vi "IMAQController.CalculateOverlay.vi"(1 "activatedCameras":T2(array[cluster]), 2 "Select Camera":u16(ring) items=["HITRAP TR1DF0", "HITRAP TR1DF2"], 6 "Line Every mm":dbl=10.0) -> (16 "Overlay Lines":T3(array[cluster]), 18 "Error?":bool)   [LabVIEW 2014, in "IMAQController.lvlib"]
uses:
  IMAQController.lvlib
  <vilib>/Utility/miscctls.llb/LVPoint32TypeDef.ctl
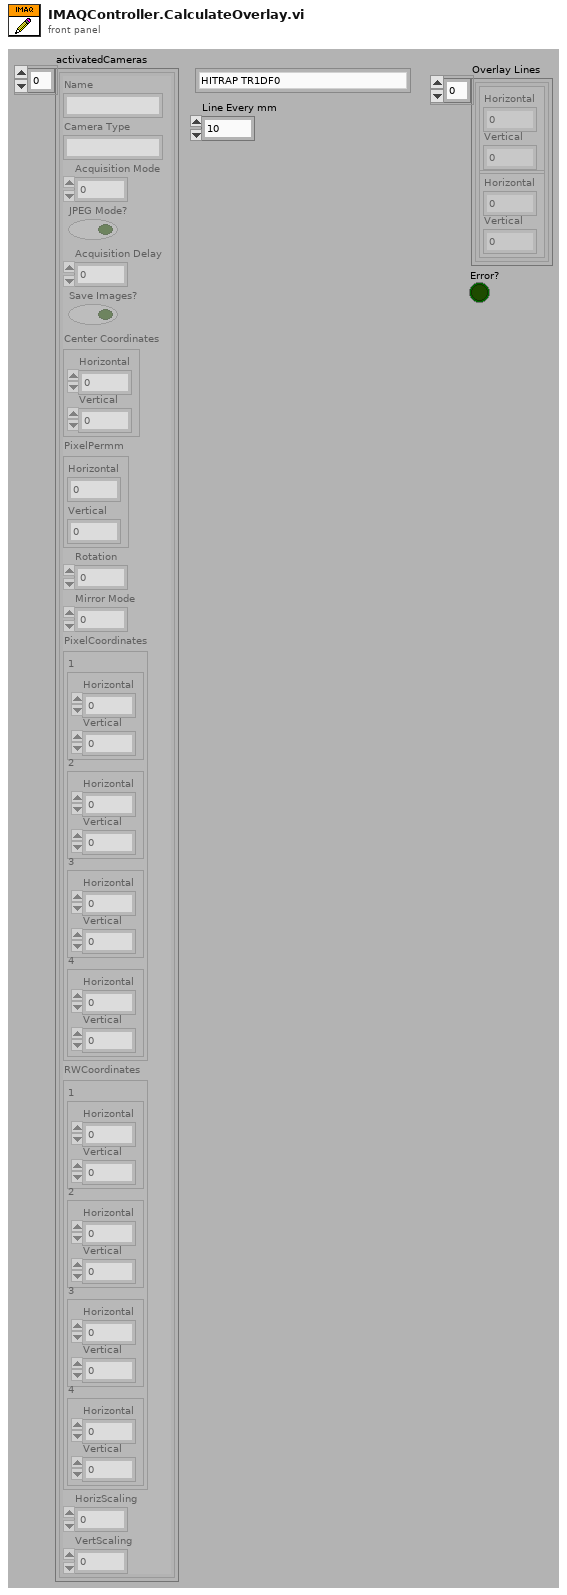
[diagram p1: front panel]
types:
  T1 = typedef "LVPoint32TypeDef.ctl" = cluster{"Horizontal":i32, "Vertical":i32}
  T2 = cluster{"Name":string, "Camera Type":string, "Acquisition Mode":u32, "JPEG Mode?":bool, "Acquisition Delay":dbl, "Save Images?":bool, "Center Coordinates":T1, "PixelPermm":cluster{"Horizontal":dbl, "Vertical":dbl}, "Rotation":dbl, "Mirror Mode":u32, "PixelCoordinates":cluster{"1":cluster{"Horizontal":i32, "Vertical":i32}, "2":cluster{"Horizontal":i32, "Vertical":i32}, "3":cluster{"Horizontal":i32, "Vertical":i32}, "4":cluster{"Horizontal":i32, "Vertical":i32}}, "RWCoordinates":cluster{"1":cluster{"Horizontal":dbl, "Vertical":dbl}, "2":cluster{"Horizontal":dbl, "Vertical":dbl}, "3":cluster{"Horizontal":dbl, "Vertical":dbl}, "4":cluster{"Horizontal":dbl, "Vertical":dbl}}, "HorizScaling":dbl, "VertScaling":dbl}[]
  T3 = cluster{cluster{"Horizontal":i32, "Vertical":i32}, cluster{"Horizontal":i32, "Vertical":i32}}[]
  T4 = cluster{"Name":string, "Camera Type":string, "Acquisition Mode":u32, "JPEG Mode?":bool, "Acquisition Delay":dbl, "Save Images?":bool, "Center Coordinates":T1, "PixelPermm":cluster{"Horizontal":dbl, "Vertical":dbl}, "Rotation":dbl, "Mirror Mode":u32, "PixelCoordinates":cluster{"1":cluster{"Horizontal":i32, "Vertical":i32}, "2":cluster{"Horizontal":i32, "Vertical":i32}, "3":cluster{"Horizontal":i32, "Vertical":i32}, "4":cluster{"Horizontal":i32, "Vertical":i32}}, "RWCoordinates":cluster{"1":cluster{"Horizontal":dbl, "Vertical":dbl}, "2":cluster{"Horizontal":dbl, "Vertical":dbl}, "3":cluster{"Horizontal":dbl, "Vertical":dbl}, "4":cluster{"Horizontal":dbl, "Vertical":dbl}}, "HorizScaling":dbl, "VertScaling":dbl}
  T5 = cluster{"1":cluster{"Horizontal":i32, "Vertical":i32}, "2":cluster{"Horizontal":i32, "Vertical":i32}, "3":cluster{"Horizontal":i32, "Vertical":i32}, "4":cluster{"Horizontal":i32, "Vertical":i32}}
  T6 = cluster{"1":cluster{"Horizontal":dbl, "Vertical":dbl}, "2":cluster{"Horizontal":dbl, "Vertical":dbl}, "3":cluster{"Horizontal":dbl, "Vertical":dbl}, "4":cluster{"Horizontal":dbl, "Vertical":dbl}}
  T7 = cluster{cluster{"Horizontal":i32, i32}, cluster{"Horizontal":i32, i32}}
  T8 = cluster{cluster{i32, "Vertical":i32}, cluster{i32, "Vertical":i32}}
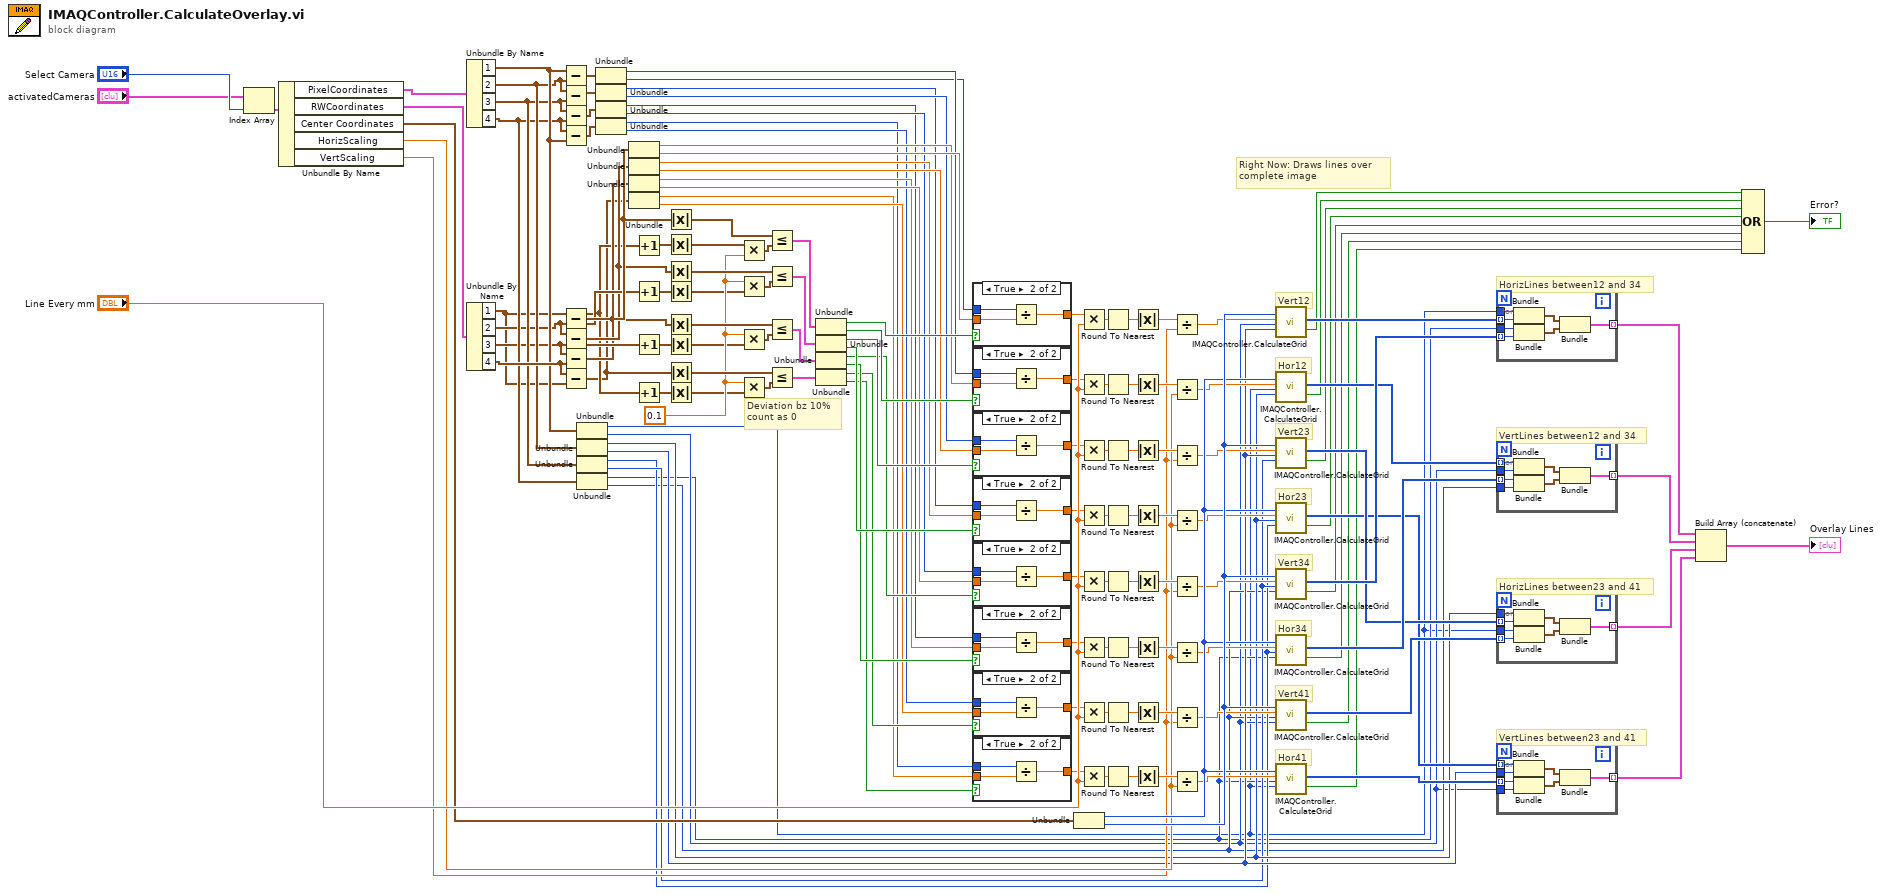
[diagram p0: block diagram]
diagram:
  w32 = 0.1
  # "Deviation bz 10% \ncount as 0"
  # "VertLines between23 and 41"
  # "HorizLines between23 and 41"
  # "VertLines between12 and 34"
  # "HorizLines between12 and 34"
  # "Right Now: Draws lines over \ncomplete image"
  # "Hor41"
  # "Vert41"
  # "Hor34"
  # "Vert34"
  # "Hor23"
  # "Vert23"
  # "Hor12"
  # "Vert12"
  n1 = Index Array(array="activatedCameras", index="Select Camera") -> (element=w140:T4)
  n2 = Unbundle By Name(w140) -> ("PixelCoordinates"=w138:T5, "RWCoordinates"=w139:T6, "Center Coordinates"=w102:T1, "HorizScaling"=w49:dbl, "VertScaling"=w48:dbl)
  n3 = Unbundle By Name(w138) -> ("1"=w82:cluster{"Horizontal":i32, "Vertical":i32}, "2"=w81:cluster{"Horizontal":i32, "Vertical":i32}, "3"=w80:cluster{"Horizontal":i32, "Vertical":i32}, "4"=w79:cluster{"Horizontal":i32, "Vertical":i32})
  n4 = Unbundle By Name(w139) -> ("1"=w10:cluster{"Horizontal":dbl, "Vertical":dbl}, "2"=w14:cluster{"Horizontal":dbl, "Vertical":dbl}, "3"=w12:cluster{"Horizontal":dbl, "Vertical":dbl}, "4"=w83:cluster{"Horizontal":dbl, "Vertical":dbl})
  n5 = Subtract(x=w82, y=w81) -> (x-y=w129:cluster{"Horizontal":i32, "Vertical":i32})
  n6 = Subtract(x=w81, y=w80) -> (x-y=w128:cluster{"Horizontal":i32, "Vertical":i32})
  n7 = Subtract(x=w80, y=w79) -> (x-y=w127:cluster{"Horizontal":i32, "Vertical":i32})
  n8 = Subtract(x=w79, y=w82) -> (x-y=w126:cluster{"Horizontal":i32, "Vertical":i32})
  n9 = Subtract(x=w10, y=w14) -> (x-y=w15:cluster{"Horizontal":dbl, "Vertical":dbl})
  n10 = Subtract(x=w14, y=w12) -> (x-y=w13:cluster{"Horizontal":dbl, "Vertical":dbl})
  n11 = Subtract(x=w12, y=w83) -> (x-y=w11:cluster{"Horizontal":dbl, "Vertical":dbl})
  n12 = Subtract(x=w83, y=w10) -> (x-y=w9:cluster{"Horizontal":dbl, "Vertical":dbl})
  n13 = Unbundle(w82) -> ("Horizontal"=w39:i32, "Vertical"=w41:i32)
  n14 = Unbundle(w81) -> ("Horizontal"=w45:i32, "Vertical"=w46:i32)
  n15 = Unbundle(w80) -> ("Horizontal"=w43:i32, "Vertical"=w44:i32)
  n16 = Unbundle(w79) -> ("Horizontal"=w40:i32, "Vertical"=w42:i32)
  n17 = Unbundle(w129) -> ("Horizontal"=w124:i32, "Vertical"=w47:i32)
  n18 = Unbundle(w128) -> ("Horizontal"=w120:i32, "Vertical"=w122:i32)
  n19 = Unbundle(w127) -> ("Horizontal"=w116:i32, "Vertical"=w118:i32)
  n20 = Unbundle(w126) -> ("Horizontal"=w112:i32, "Vertical"=w114:i32)
  n21 = Unbundle(w15) -> ("Horizontal"=w123:dbl, "Vertical"=w125:dbl)
  n22 = Unbundle(w13) -> ("Horizontal"=w119:dbl, "Vertical"=w121:dbl)
  n23 = Unbundle(w11) -> ("Horizontal"=w115:dbl, "Vertical"=w117:dbl)
  n24 = Unbundle(w9) -> ("Horizontal"=w111:dbl, "Vertical"=w113:dbl)
  n25 = Increment(x=w10) -> (x+1=w8:cluster{"Horizontal":dbl, "Vertical":dbl})
  n26 = Increment(x=w14) -> (x+1=w6:cluster{"Horizontal":dbl, "Vertical":dbl})
  n27 = Increment(x=w12) -> (x+1=w3:cluster{"Horizontal":dbl, "Vertical":dbl})
  n28 = Increment(x=w10) -> (x+1=w1:cluster{"Horizontal":dbl, "Vertical":dbl})
  n29 = Absolute Value(x=w15) -> (abs(x)=w37:cluster{"Horizontal":dbl, "Vertical":dbl})
  n30 = Absolute Value(x=w8) -> (abs(x)=w7:cluster{"Horizontal":dbl, "Vertical":dbl})
  n31 = Absolute Value(x=w13) -> (abs(x)=w35:cluster{"Horizontal":dbl, "Vertical":dbl})
  n32 = Absolute Value(x=w6) -> (abs(x)=w5:cluster{"Horizontal":dbl, "Vertical":dbl})
  n33 = Absolute Value(x=w11) -> (abs(x)=w34:cluster{"Horizontal":dbl, "Vertical":dbl})
  n34 = Absolute Value(x=w3) -> (abs(x)=w4:cluster{"Horizontal":dbl, "Vertical":dbl})
  n35 = Absolute Value(x=w9) -> (abs(x)=w33:cluster{"Horizontal":dbl, "Vertical":dbl})
  n36 = Absolute Value(x=w1) -> (abs(x)=w2:cluster{"Horizontal":dbl, "Vertical":dbl})
  n37 = Multiply(x=w7, y=w32) -> (x*y=w16:cluster{"Horizontal":dbl, "Vertical":dbl})
  n38 = Multiply(x=w32, y=w5) -> (x*y=w17:cluster{"Horizontal":dbl, "Vertical":dbl})
  n39 = Multiply(x=w32, y=w4) -> (x*y=w18:cluster{"Horizontal":dbl, "Vertical":dbl})
  n40 = Multiply(x=w32, y=w2) -> (x*y=w19:cluster{"Horizontal":dbl, "Vertical":dbl})
  n41 = Less Or Equal?(x=w37, y=w16) -> (x <= y?=w36:cluster{"Horizontal":bool, "Vertical":bool})
  n42 = Less Or Equal?(x=w35, y=w17) -> (x <= y?=w31:cluster{"Horizontal":bool, "Vertical":bool})
  n43 = Less Or Equal?(x=w34, y=w18) -> (x <= y?=w30:cluster{"Horizontal":bool, "Vertical":bool})
  n44 = Less Or Equal?(x=w33, y=w19) -> (x <= y?=w29:cluster{"Horizontal":bool, "Vertical":bool})
  n45 = Unbundle(w36) -> ("Horizontal"=w137:bool, "Vertical"=w136:bool)
  n46 = Unbundle(w31) -> ("Horizontal"=w135:bool, "Vertical"=w134:bool)
  n47 = Unbundle(w30) -> ("Horizontal"=w133:bool, "Vertical"=w132:bool)
  n48 = Unbundle(w29) -> ("Horizontal"=w131:bool, "Vertical"=w130:bool)
  n49 = case shown="True" w137 {
    tunnel: w47 -> [_ w145]
    tunnel: w125 -> [_ w144]
    tunnel: [_ w143] -> w110
    frame False {
    }
    frame True {
      n50 = Divide(x=w145, y=w144) -> (x/y=w143:dbl)
    }
  }
  n51 = case shown="True" w136 {
    tunnel: [_ w148] -> w109
    tunnel: w124 -> [_ w147]
    tunnel: w123 -> [_ w146]
    frame False {
    }
    frame True {
      n52 = Divide(x=w147, y=w146) -> (x/y=w148:dbl)
    }
  }
  n53 = case shown="True" w135 {
    tunnel: [_ w151] -> w108
    tunnel: w122 -> [_ w150]
    tunnel: w121 -> [_ w149]
    frame False {
    }
    frame True {
      n54 = Divide(x=w150, y=w149) -> (x/y=w151:dbl)
    }
  }
  n55 = case shown="True" w134 {
    tunnel: [_ w154] -> w107
    tunnel: w120 -> [_ w153]
    tunnel: w119 -> [_ w152]
    frame False {
    }
    frame True {
      n56 = Divide(x=w153, y=w152) -> (x/y=w154:dbl)
    }
  }
  n57 = case shown="True" w133 {
    tunnel: [_ w157] -> w106
    tunnel: w118 -> [_ w156]
    tunnel: w117 -> [_ w155]
    frame False {
    }
    frame True {
      n58 = Divide(x=w156, y=w155) -> (x/y=w157:dbl)
    }
  }
  n59 = case shown="True" w132 {
    tunnel: [_ w160] -> w105
    tunnel: w116 -> [_ w159]
    tunnel: w115 -> [_ w158]
    frame False {
    }
    frame True {
      n60 = Divide(x=w159, y=w158) -> (x/y=w160:dbl)
    }
  }
  n61 = case shown="True" w131 {
    tunnel: [_ w163] -> w104
    tunnel: w114 -> [_ w162]
    tunnel: w113 -> [_ w161]
    frame False {
    }
    frame True {
      n62 = Divide(x=w162, y=w161) -> (x/y=w163:dbl)
    }
  }
  n63 = case shown="True" w130 {
    tunnel: [_ w166] -> w103
    tunnel: w112 -> [_ w165]
    tunnel: w111 -> [_ w164]
    frame False {
    }
    frame True {
      n64 = Divide(x=w165, y=w164) -> (x/y=w166:dbl)
    }
  }
  n65 = Unbundle(w102) -> ("Horizontal"=w92:i32, "Vertical"=w93:i32)
  n66 = Multiply(x=w110, y="Line Every mm") -> (x*y=w101:dbl)
  n67 = Multiply(x=w109, y="Line Every mm") -> (x*y=w100:dbl)
  n68 = Multiply(x=w108, y="Line Every mm") -> (x*y=w99:dbl)
  n69 = Multiply(x=w107, y="Line Every mm") -> (x*y=w98:dbl)
  n70 = Multiply(x=w106, y="Line Every mm") -> (x*y=w97:dbl)
  n71 = Multiply(x=w105, y="Line Every mm") -> (x*y=w96:dbl)
  n72 = Multiply(x=w104, y="Line Every mm") -> (x*y=w95:dbl)
  n73 = Multiply(x=w103, y="Line Every mm") -> (x*y=w94:dbl)
  n74 = Round To Nearest(number=w101) -> (nearest integer value=w73:dbl)
  n75 = Round To Nearest(number=w100) -> (nearest integer value=w72:dbl)
  n76 = Round To Nearest(number=w99) -> (nearest integer value=w71:dbl)
  n77 = Round To Nearest(number=w98) -> (nearest integer value=w70:dbl)
  n78 = Round To Nearest(number=w97) -> (nearest integer value=w69:dbl)
  n79 = Round To Nearest(number=w96) -> (nearest integer value=w68:dbl)
  n80 = Round To Nearest(number=w95) -> (nearest integer value=w67:dbl)
  n81 = Round To Nearest(number=w94) -> (nearest integer value=w66:dbl)
  n82 = Absolute Value(x=w73) -> (abs(x)=w65:dbl)
  n83 = Absolute Value(x=w72) -> (abs(x)=w63:dbl)
  n84 = Absolute Value(x=w71) -> (abs(x)=w61:dbl)
  n85 = Absolute Value(x=w70) -> (abs(x)=w59:dbl)
  n86 = Absolute Value(x=w69) -> (abs(x)=w56:dbl)
  n87 = Absolute Value(x=w68) -> (abs(x)=w54:dbl)
  n88 = Absolute Value(x=w67) -> (abs(x)=w53:dbl)
  n89 = Absolute Value(x=w66) -> (abs(x)=w51:dbl)
  n90 = Divide(x=w65, y=w48) -> (x/y=w64:dbl)
  n91 = Divide(x=w63, y=w49) -> (x/y=w62:dbl)
  n92 = Divide(x=w61, y=w48) -> (x/y=w60:dbl)
  n93 = Divide(x=w59, y=w49) -> (x/y=w58:dbl)
  n94 = Divide(x=w56, y=w48) -> (x/y=w57:dbl)
  n95 = Divide(x=w54, y=w49) -> (x/y=w55:dbl)
  n96 = Divide(x=w53, y=w48) -> (x/y=w52:dbl)
  n97 = Divide(x=w51, y=w49) -> (x/y=w50:dbl)
  n98 = call "IMAQController.CalculateGrid.vi"("Central"=w93, "PixelDistanceBetweenGridLines"=w64, "AxesMin"=w41, "AxesMax"=w46) -> ("sorted array"=w91:i32[], "Error"=w28:bool)  [unwired: 14 in]
  n99 = call "IMAQController.CalculateGrid.vi"("Central"=w92, "PixelDistanceBetweenGridLines"=w62, "AxesMin"=w39, "AxesMax"=w45) -> ("sorted array"=w89:i32[], "Error"=w27:bool)  [unwired: 14 in]
  n100 = call "IMAQController.CalculateGrid.vi"("Central"=w93, "PixelDistanceBetweenGridLines"=w60, "AxesMin"=w46, "AxesMax"=w44) -> ("sorted array"=w87:i32[], "Error"=w26:bool)  [unwired: 14 in]
  n101 = call "IMAQController.CalculateGrid.vi"("Central"=w92, "PixelDistanceBetweenGridLines"=w58, "AxesMin"=w45, "AxesMax"=w43) -> ("sorted array"=w84:i32[], "Error"=w25:bool)  [unwired: 14 in]
  n102 = call "IMAQController.CalculateGrid.vi"("Central"=w93, "PixelDistanceBetweenGridLines"=w57, "AxesMin"=w44, "AxesMax"=w42) -> ("sorted array"=w90:i32[], "Error"=w24:bool)  [unwired: 14 in]
  n103 = call "IMAQController.CalculateGrid.vi"("Central"=w92, "PixelDistanceBetweenGridLines"=w55, "AxesMin"=w43, "AxesMax"=w40) -> ("sorted array"=w88:i32[], "Error"=w23:bool)  [unwired: 14 in]
  n104 = call "IMAQController.CalculateGrid.vi"("Central"=w93, "PixelDistanceBetweenGridLines"=w52, "AxesMin"=w42, "AxesMax"=w41) -> ("sorted array"=w86:i32[], "Error"=w22:bool)  [unwired: 14 in]
  n105 = call "IMAQController.CalculateGrid.vi"("Central"=w92, "PixelDistanceBetweenGridLines"=w50, "AxesMin"=w40, "AxesMax"=w39) -> ("sorted array"=w85:i32[], "Error"=w21:bool)  [unwired: 14 in]
  n106 = for {
    tunnel: [w171] -> w78 mode=indexing
    tunnel: w91 -> [w170] mode=indexing
    tunnel: w39 -> [w169]
    tunnel: w40 -> [w168]
    tunnel: w90 -> [w167] mode=indexing
    n107 = Bundle("Horizontal"=w169, w170) -> (w172:cluster{"Horizontal":i32, i32})  [unwired: 1 in]
    n108 = Bundle("Horizontal"=w168, w167) -> (w173:cluster{"Horizontal":i32, i32})  [unwired: 1 in]
    n109 = Bundle(w172, w173) -> (w171:T7)  [unwired: 1 in]
  }
  n110 = for {
    tunnel: [w178] -> w77 mode=indexing
    tunnel: w89 -> [w177] mode=indexing
    tunnel: w88 -> [w176] mode=indexing
    tunnel: w41 -> [w175]
    tunnel: w42 -> [w174]
    n111 = Bundle(w177, "Vertical"=w175) -> (w179:cluster{i32, "Vertical":i32})  [unwired: 1 in]
    n112 = Bundle(w176, "Vertical"=w174) -> (w180:cluster{i32, "Vertical":i32})  [unwired: 1 in]
    n113 = Bundle(w179, w180) -> (w178:T8)  [unwired: 1 in]
  }
  n114 = for {
    tunnel: [w185] -> w76 mode=indexing
    tunnel: w87 -> [w184] mode=indexing
    tunnel: w86 -> [w183] mode=indexing
    tunnel: w45 -> [w182]
    tunnel: w39 -> [w181]
    n115 = Bundle("Horizontal"=w182, w184) -> (w186:cluster{"Horizontal":i32, i32})  [unwired: 1 in]
    n116 = Bundle("Horizontal"=w181, w183) -> (w187:cluster{"Horizontal":i32, i32})  [unwired: 1 in]
    n117 = Bundle(w186, w187) -> (w185:T7)  [unwired: 1 in]
  }
  n118 = for {
    tunnel: [w192] -> w75 mode=indexing
    tunnel: w85 -> [w191] mode=indexing
    tunnel: w84 -> [w190] mode=indexing
    tunnel: w46 -> [w189]
    tunnel: w41 -> [w188]
    n119 = Bundle(w190, "Vertical"=w189) -> (w193:cluster{i32, "Vertical":i32})  [unwired: 1 in]
    n120 = Bundle(w191, "Vertical"=w188) -> (w194:cluster{i32, "Vertical":i32})  [unwired: 1 in]
    n121 = Bundle(w193, w194) -> (w192:T8)  [unwired: 1 in]
  }
  n122 = Build Array (concatenate)(w78, w77, w76, w75) -> (→"Overlay Lines":T3)
  n123 = Compound Arithmetic op=OR(w28, w27, w26, w25, w24, w23, w22, w21) -> (→"Error?":bool)
